vi "Update Data Rate.vi"(8 "error in":errorcluster, 10 "Rate":dbl, 11 "objects":T1) -> (0 "error out":errorcluster)   [LabVIEW 2014, in "DAQmx Module Editor Node.lvclass"]
uses:
  DAQmx Module Editor Node.lvclass
  <vilib>/NI/DCAF/Tag Editor Core/Table API/Table Manager/object ref.ctl
  <vilib>/NI/DCAF/Tag Editor Core/Configuration Editor/Classes/Engine Parent/Engine Parent Editor Node.lvclass
  <vilib>/NI/DCAF/Tag Editor Core/Configuration Editor/Classes/Module editor node/module editor node.lvclass
  module/configuration/DAQmx Module Configuration.lvclass
  module/configuration/Write Data Rate.vi
  <vilib>/NI/Configuration Framework/serializable configuration/NISE_CEF_serializable configuration.lvclass
  <vilib>/NI/DCAF/Tag Editor Core/Table API/Table Manager/Table Manager.lvclass
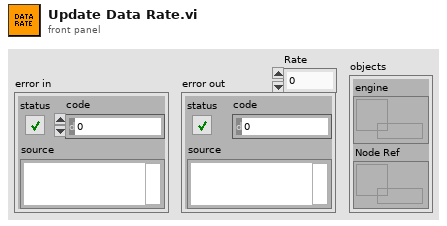
[diagram p1: front panel]
types:
  T1 = typedef "Table Manager.lvlib/Table Manager.lvclass/object ref.ctl" = cluster{"engine":refnum<data-value>, "Node Ref":refnum<data-value>}
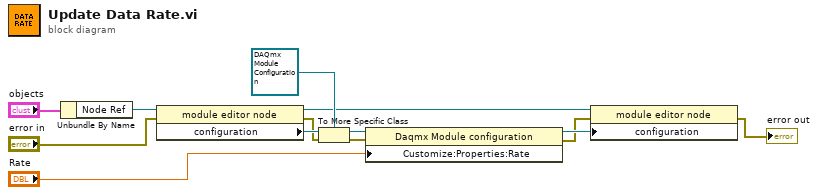
[diagram p0: block diagram]
diagram:
  n1 = Unbundle By Name("objects") -> ("Node Ref"=w4:refnum<data-value>)
  n2 = property class="module editor node"(reference=w4, error in="error in") -> (reference out=w3:refnum<data-value>, error out=w7:errorcluster, "configuration"=w11:refnum<class "NISE_CEF_serializable configuration.lvclass">)
  n3 = To More Specific Class(target class=refnum<class "DAQmx Module Configuration.lvclass"> refnum ("tag bus configurable plugin module configuration"), reference=w11, error in=w7) -> (specific class reference=w8:refnum<class "DAQmx Module Configuration.lvclass">, error out=w6:errorcluster)
  n4 = property class="Daqmx Module configuration"(reference=w8, error in=w6, "Customize:Properties:Rate"="Rate") -> (reference out=w5:refnum<class "DAQmx Module Configuration.lvclass">, error out=w2:errorcluster)
  n5 = property class="module editor node"(reference=w3, error in=w2, "configuration"=w5) -> (error out=→"error out":errorcluster)  [unwired: 1 out]
